vi "SubPanel_PowerConfiguration_Rev11_v2.vi"(8 "error in":errorcluster, 10 "VISAPowerInfoInputArray":T2(array[cluster]), 11 "DCPowerInformationClusterArray_Input":T1(array[cluster])) -> (0 "error out":errorcluster, 2 "VISAPowerInfoOutputArray":T2(array[cluster]), 3 "DCPowerInformationClusterArray_Output":T1(array[cluster]))   [LabVIEW 2019]
panel:
  out "DCPowerInformationClusterArray":T1(array[cluster])
  in  "Update Changes (MUST HAVE ACTIVE CHANNEL SELECTED FOR CHANGES TO BE APPLIED)":bool
  out "VISAPowerInformationClusterArray":T2(array[cluster])
  out "VISAPowerInformationClusterOutput":T3(array[cluster])
  in  "VISAPowerInformationClusterInput":T3(array[cluster])
  in  "Exit SubVI":bool
  in  "Instrument Cards (Must Reconfigure if you add new cards or change the names in NI Max)":T4(tab)=enum."PXIe-4139"
  in  "VISA resource name":refnum<visa-resource-name>
  in  "Apply Power Settings":bool
  out "POWER STATUS":bool
  in  "POWER ON":bool
  in  "Voltage Channel 1":dbl
  in  "Voltage Channel 2":dbl
  in  "Voltage Channel 3":dbl
  in  "Current Limit Channel 1":dbl
  in  "Current Limit Channel 2":dbl
  in  "Current Limit Channel 3":dbl
  out "Parameter Configuration Echo":string[][](array[string])
  out "Configuration Echo":string
  in  "Which Channels to Parallelize":u16(ring) items=["I1+I2", "ALL", "I2+I3"]
  in  "Combination Scheme":u16(ring) items=["OFF", "SERIES", "PARALLEL"]
  in  "voltage level channel 0":dbl format="%.6p"
  in  "voltage level channel 1":dbl format="%.6p"
  in  "voltage level channel 2":dbl format="%.6p"
  in  "voltage level channel 3":dbl format="%.6p"
  in  "voltage level channel 4":dbl format="%.6p"
  in  "voltage level channel 5":dbl format="%.6p"
  in  "voltage level channel 6":dbl format="%.6p"
  in  "voltage level channel 7":dbl format="%.6p"
  in  "voltage level channel 8":dbl format="%.6p"
  in  "voltage level channel 9":dbl format="%.6p"
  in  "voltage level channel 10":dbl format="%.6p"
  in  "voltage level channel 11":dbl format="%.6p"
  in  "voltage level channel 12":dbl format="%.6p"
  in  "voltage level channel 13":dbl format="%.6p"
  in  "voltage level channel 14":dbl format="%.6p"
  in  "voltage level channel 15":dbl format="%.6p"
  in  "voltage level channel 16":dbl format="%.6p"
  in  "voltage level channel 17":dbl format="%.6p"
  in  "voltage level channel 18":dbl format="%.6p"
  in  "voltage level channel 19":dbl format="%.6p"
  in  "voltage level channel 20":dbl format="%.6p"
  in  "voltage level channel 21":dbl format="%.6p"
  in  "voltage level channel 22":dbl format="%.6p"
  in  "voltage level channel 23":dbl format="%.6p"
  in  "Active Channel 0":bool
  in  "Active Channel 1":bool
  in  "Active Channel 2":bool
  in  "Active Channel 3":bool
  in  "Active Channel 4":bool
  in  "Active Channel 5":bool
  in  "Active Channel 6":bool
  in  "Active Channel 7":bool
  in  "Active Channel 8":bool
  in  "Active Channel 9":bool
  in  "Active Channel 10":bool
  in  "Active Channel 11":bool
  in  "Active Channel 12":bool
  in  "Active Channel 13":bool
  in  "Active Channel 14":bool
  in  "Active Channel 15":bool
  in  "Active Channel 16":bool
  in  "Active Channel 17":bool
  in  "Active Channel 18":bool
  in  "Active Channel 19":bool
  in  "Active Channel 20":bool
  in  "Active Channel 21":bool
  in  "Active Channel 22":bool
  in  "Active Channel 23":bool
  in  "Channel Name 0":string="NULL0"
  in  "Channel Name 1":string="1p8V_supply"
  in  "Channel Name 2":string="NULL2"
  in  "Channel Name 3":string="NULL3"
  in  "Channel Name 4":string="NULL4"
  in  "Channel Name 5":string="NULL5"
  in  "Channel Name 6":string="NULL6"
  in  "Channel Name 7":string="NULL7"
  in  "Channel Name 8":string="NULL8"
  in  "Channel Name 9":string="NULL9"
  in  "Channel Name 10":string="NULL10"
  in  "Channel Name 11":string="NULL11"
  in  "Channel Name 12":string="NULL12"
  in  "Channel Name 13":string="NULL13"
  in  "Channel Name 14":string="NULL14"
  in  "Channel Name 15":string="NULL15"
  in  "Channel Name 16":string="NULL16"
  in  "Channel Name 17":string="NULL17"
  in  "Channel Name 18":string="NULL18"
  in  "Channel Name 19":string="NULL19"
  in  "Channel Name 20":string="NULL20"
  in  "Channel Name 21":string="NULL21"
  in  "Channel Name 22":string="NULL22"
  in  "Channel Name 23":string="NULL23"
  in  "Apply Power Settings":bool
  in  "Aperture Time (s)":dbl=0.0001
  in  "Measure Record Length":i32=1000000
  in  "current limit (A)":dbl=0.05
  out "All Channel Numbers Array":string[](array[string])=["0", "1", "2", "3", "4", "5", "6", "7", "8", "9", "10", "11", "12", "13", "14", "15", "16", "17", "18", "19", "20", "21", "22", "23"]
  out "Active Channels Indicator":bool[](array[boolean])
  out "Voltage Array":dbl[](array[numeric])=[1.0, 1.8, 1.2, 1.3, 1.4, 1.5, 1.6, 1.7, 1.8, 1.9, 2.0, 2.1, 2.2, 2.3, 2.4, 2.5, 2.6, 2.7, 2.8, 2.9, 3.0, 3.1, 3.2, 3.3]
  out "Active Channel Numbers Array":string[](array[string])=["1"]
  out "Active Channel Voltage Array":dbl[](array[numeric])=[1.8]
  out "Active Channel Names Array":string[](array[string])=["1p8V_supply"]
  in  "voltage level channel 0":dbl format="%.6p"
  in  "Active Channel 0":bool
  in  "Apply Power Settings":bool
  in  "Channel Name 0":string="1p6_supply"
  out "Active Channel Voltage Array":dbl[](array[numeric])=[1.68]
  out "Active Channels Indicator":bool[](array[boolean])
  out "Voltage Array":dbl[](array[numeric])=[1.68]
  out "Active Channel Names Array":string[](array[string])=["1p6_supply"]
  out "Active Channel Numbers Array":string[](array[string])=["0"]
  out "All Channel Numbers Array":string[](array[string])=["0"]
  in  "current limit (A)":dbl=0.05
  in  "Measure Record Length":i32=1000000
  in  "Aperture Time (s)":dbl=0.001
  out "DCPowerInformationClusterOutput":T5(array[cluster])
  in  "DCPowerInformationClusterInput":T5(array[cluster])
  # "Background Information (Important)\nThis subvi has tabs that allow you to configure different power instruments. There are two options: VISA instruments or DC Power instruments. DC Power instruments are inside of the tester, visa instruments are external. If DCPower instruments are switched out, they will need to be reconfigured within the backend of this code (instructions pending). You are able to identify which channels you want to active, their individual voltage levels and the desired \"name\" of the channel (i.e. if you want channel 0 to be known at the \"ADMV1013_3p3V\" or \"GoodEnough\", you write it here). For the entire instrument, you can determine its capture rate (aperture time) or the current limit. I advise you do NOT alter the \"Measure Record Length\" as this is only if there are issues with the program. Shouldn't ever exceed this value. You apply the settings and they will be echoed back in each tab along with the array above. Multiple instruments can be configured and will show up as separate array elements\n\n\nInstructions (More Important):\n\nSelect instrument of interest (VISA KEITHLEY 2230G-30-6, PXIe-4163, and PXIe-4139 are the ones currently available). \n\n\nFOR DCPOWER INSTRUMENTS (PXI or PXIe)\n\nPress \"Active Channel #\" to select which channels you want to have power applied \n\nType in voltage level in \"Voltage level channel #\"\n\nType in desired channel name in \"Channel Name #\"\n\nType the measurement speed (suggest .0001) in aperture time\n\nType the current limit in \"current limit\"\n\nPress \"Apply Power Settings\" and review the echoed outputs within the tab and in the instrument array above the tabs.\n\nRepeat this process for other instruments\n\n\n\nFOR VISA INSTRUMENTS (NOT PXI or PXIe), note that it is case by case for instruments\n\nSelect resource name (you must know which one it is)\n\nPower on device if using it\n\nApply voltage settings \n\nApply current limits for each channel\n\nSelect which channels you will parallelize if at all\n\nSelect which combination scheme you will apply: OFF (individual channels), SERIES (Channel 1 and 2 in series), PARALLEL (I1 + I2, ALL, I2 + I3)\n\nFOR COMBINATIONS: for a combination scheme you choose, you only apply changes to the first channel of each. example: if you make the system series configuration, you only type you voltage information (i.e. 60V) into channel 1 and the current limit information into channel 1 but channel 3 is still independent of these\n\n\nPress \"Apply Powe Settings\" when complete\n\nReview the echoed values along with the instrument array above"
  # "All Voltage Level Channels are in Volts"
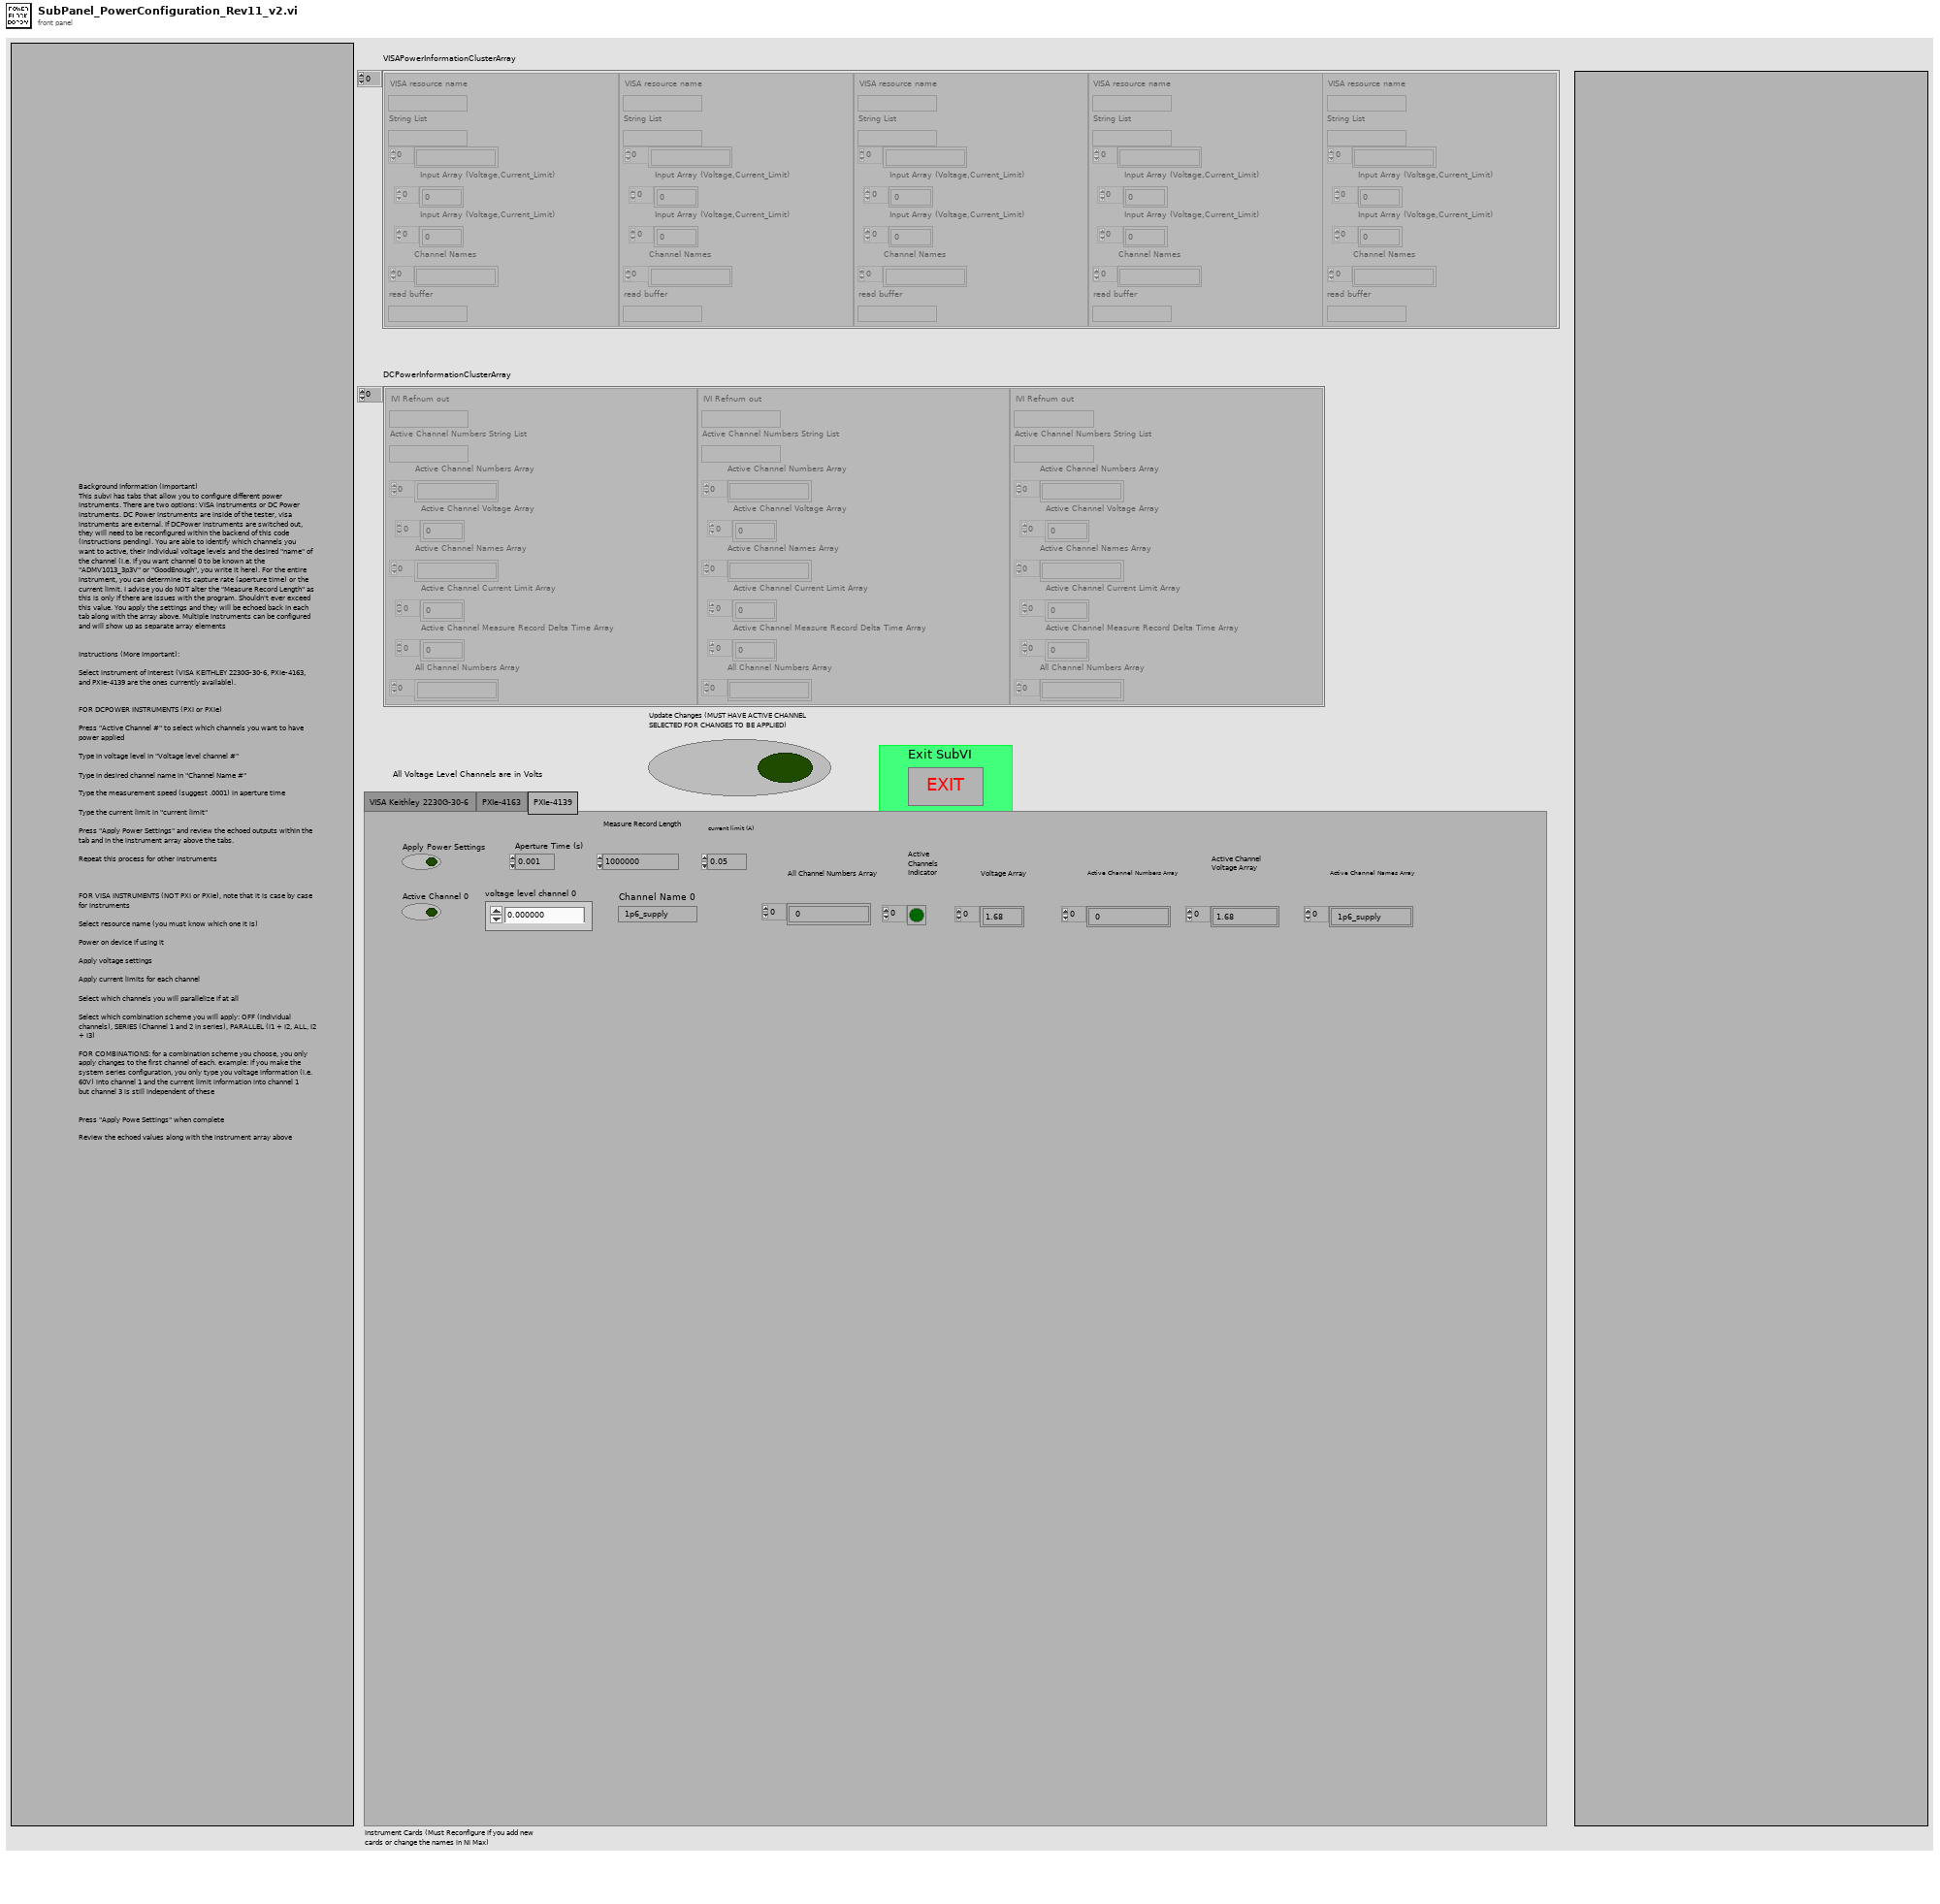
[diagram p1: front panel]
types:
  T1 = cluster{"IVI Refnum out":refnum<k15>, "Active Channel Numbers String List":string, "Active Channel Numbers Array":string[], "Active Channel Voltage Array":dbl[], "Active Channel Names Array":string[], "Active Channel Current Limit Array":dbl[], "Active Channel Measure Record Delta Time Array":dbl[], "All Channel Numbers Array":string[]}[]
  T2 = cluster{"VISA resource name":refnum<visa-resource-name>, "String List":string, string[], "Input Array (Voltage,Current_Limit)":dbl[], "Input Array (Voltage,Current_Limit)":dbl[], "Channel Names":string[], "read buffer":string}[]
  T3 = cluster{"VISA resource name":refnum<visa-resource-name>, "String List":string, string[], "Input Array (Voltage,Current_Limit)":dbl[], "Input Array (Voltage,Current_Limit)":dbl[], "Channel Names":string[]}[]
  T4 = enum32{"VISA Keithley 2230G-30-6", "PXIe-4163", "PXIe-4139"}
  T5 = cluster{"instrument handle out":refnum<k15>, string, string[], dbl[], string[]}[]
  T6 = cluster{"instrument handle out":refnum<k15>, string, string[], dbl[], string[], "Current Limit Output Array":dbl[], dbl[]}[]
  T7 = cluster{"IVI Refnum out":refnum<k15>, "Active Channel Numbers String List":string, "Active Channel Numbers Array":string[], "Active Channel Voltage Array":dbl[], "Active Channel Names Array":string[], "Active Channel Current Limit Array":dbl[], "Active Channel Measure Record Delta Time Array":dbl[], "All Channel Numbers Array":string[]}
  T8 = typedef "VISA_power_Control.ctl" = cluster{"VISA resource name":refnum<visa-resource-name>, "Active Channel List":string, "Active Channel Array":string[], "Input Array (Voltage,Current_Limit)":dbl[], "Input Array (Voltage,Current_Limit)":dbl[], "Channel Names":string[], "read buffer":string, "Channel Names Array":string[]}
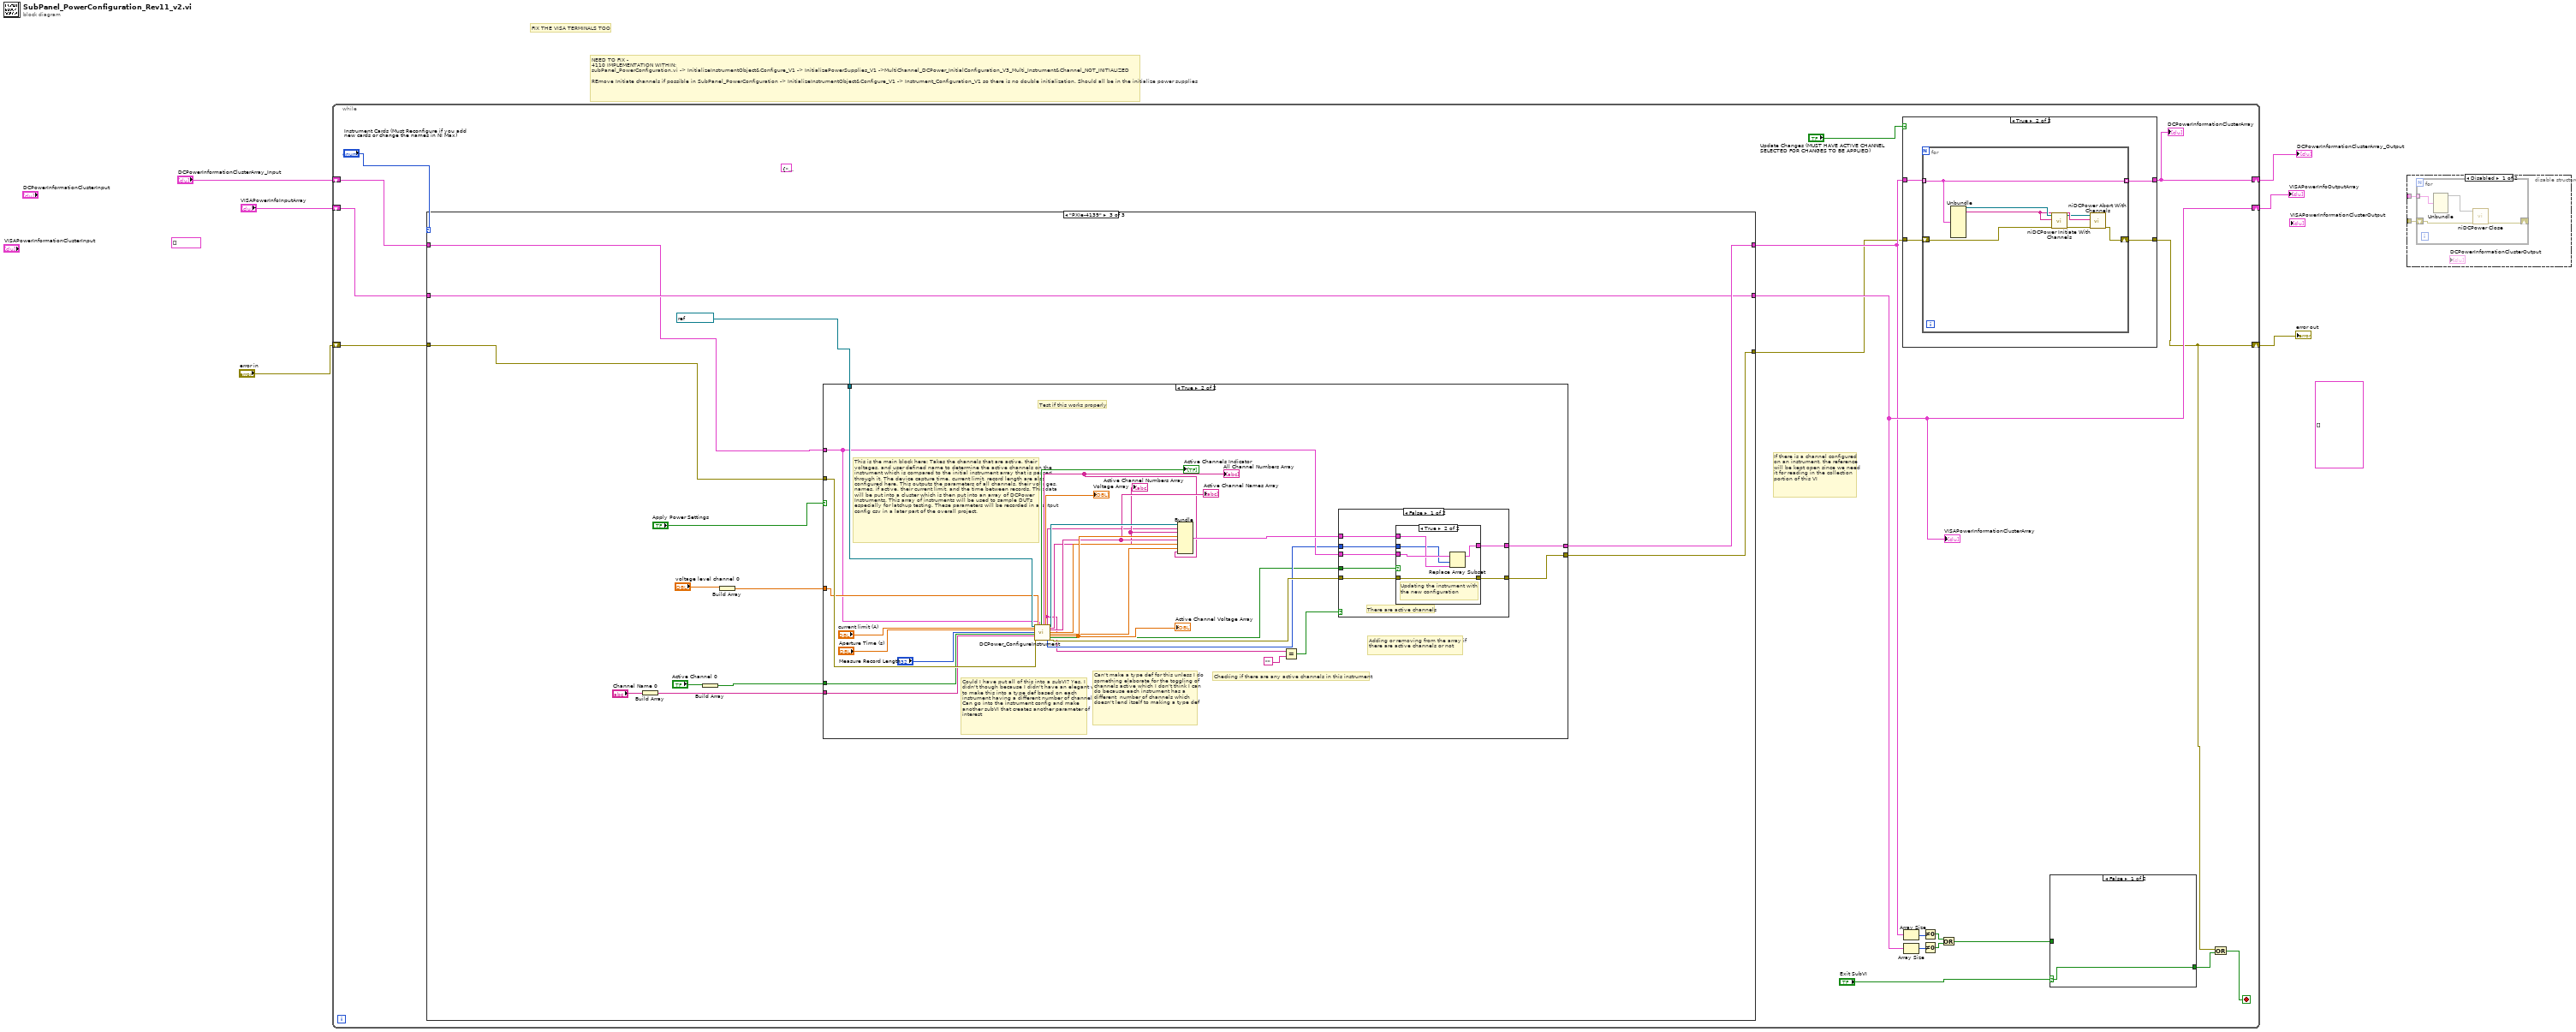
[diagram p0: block diagram]
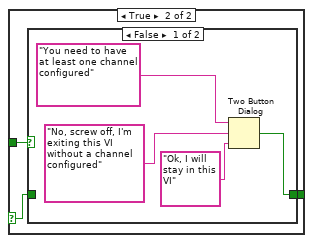
[diagram p4: hidden frame]
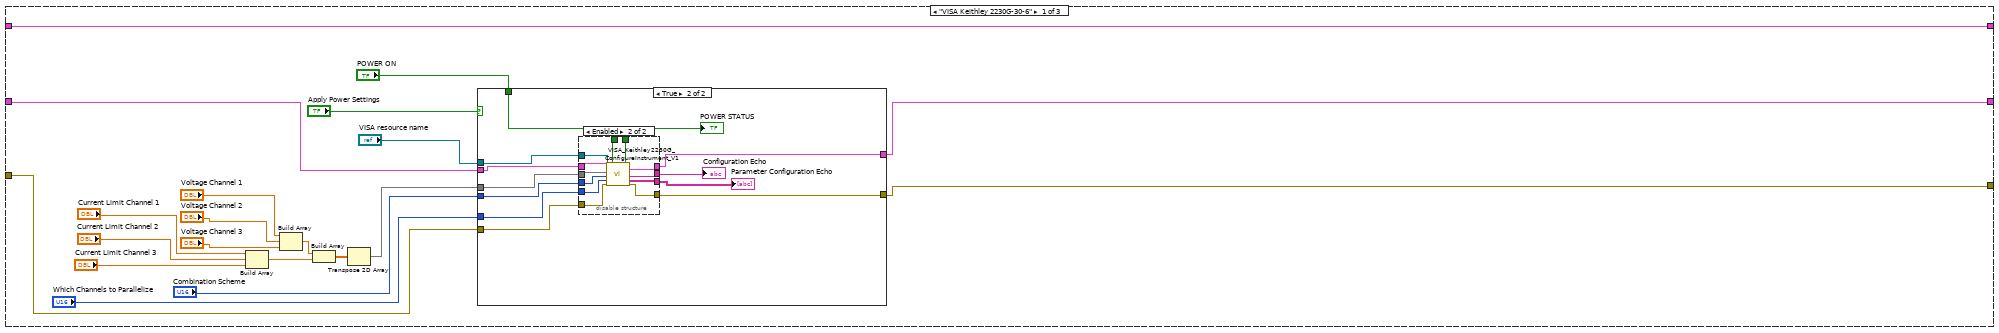
[diagram p6: hidden frame]
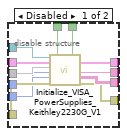
[diagram p8: hidden frame]
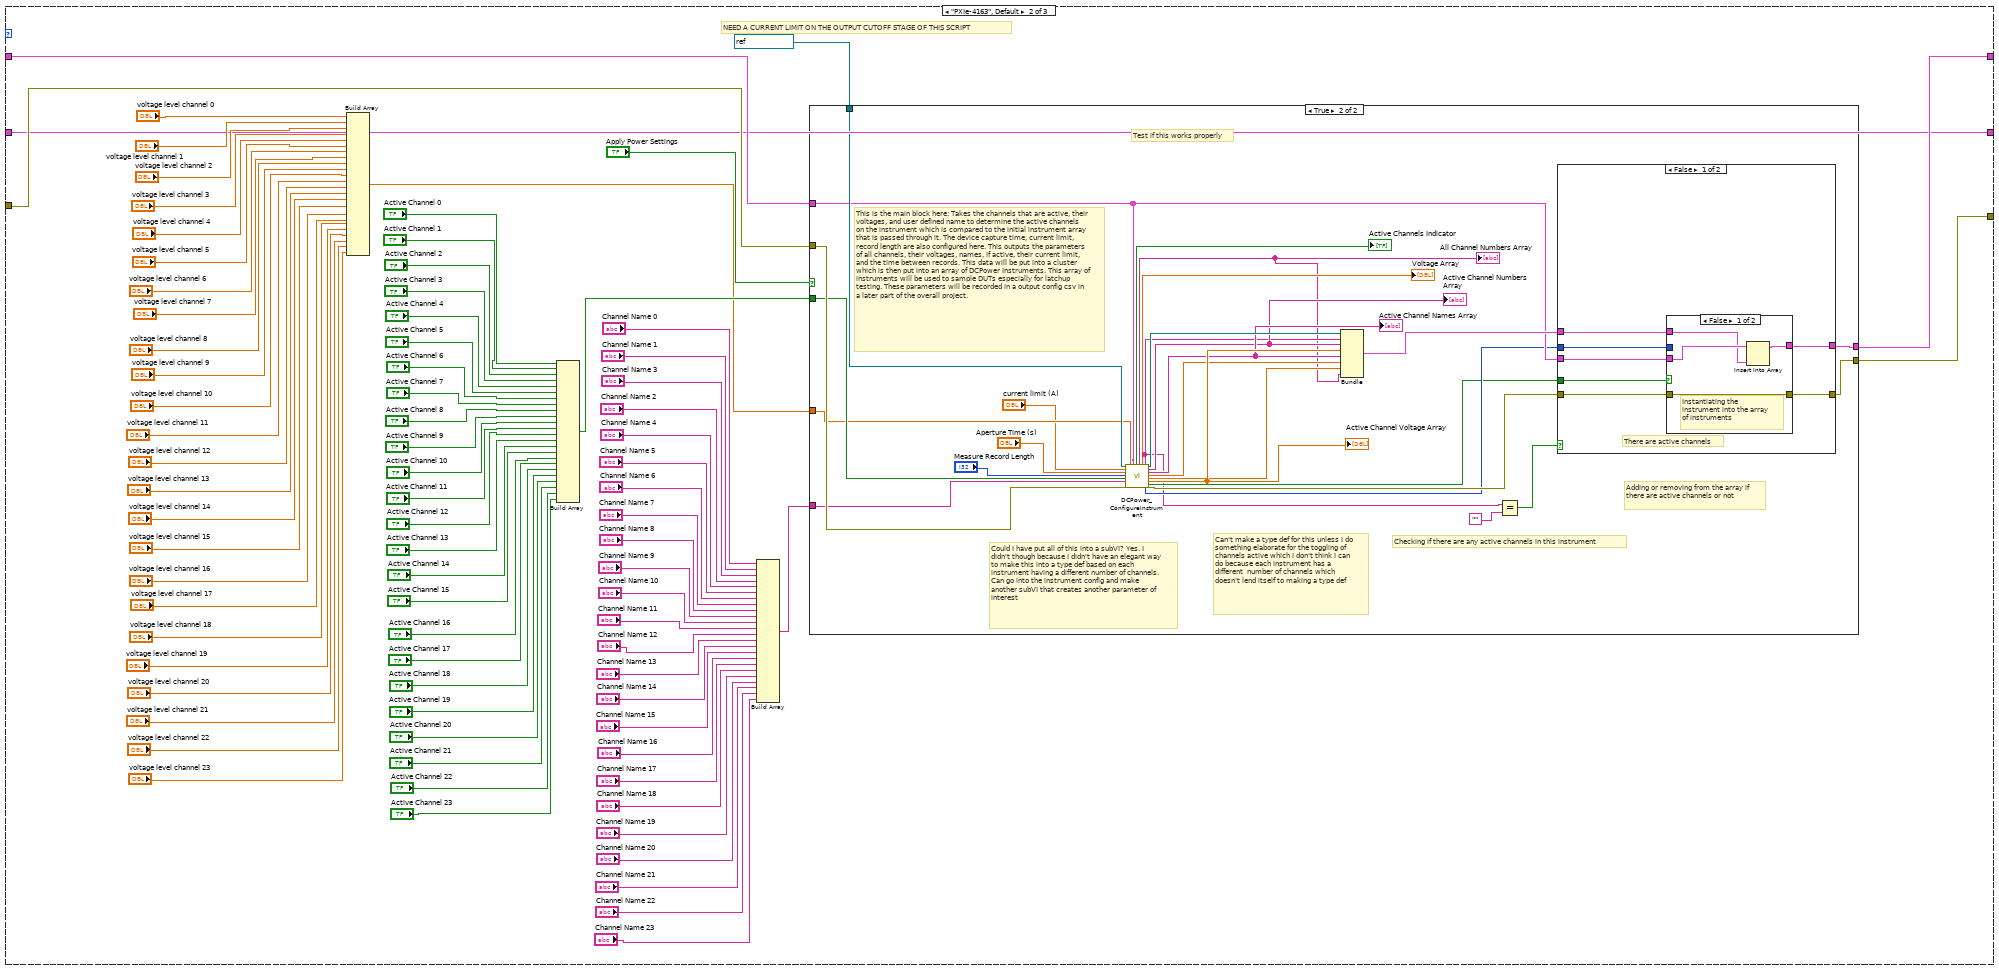
[diagram p9: hidden frame]
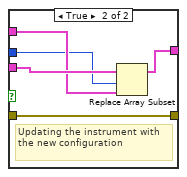
[diagram p11: hidden frame]
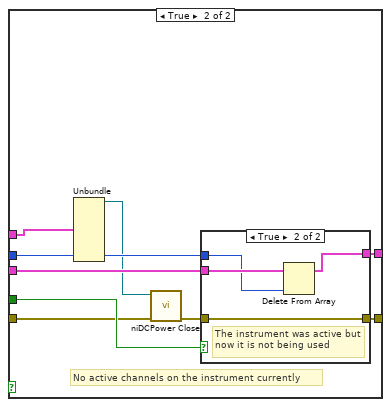
[diagram p12: hidden frame]
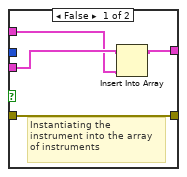
[diagram p15: hidden frame]
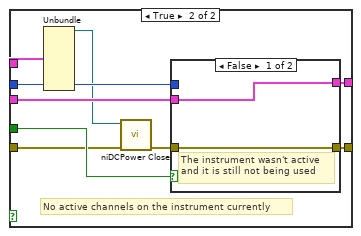
[diagram p16: hidden frame]
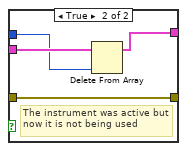
[diagram p17: hidden frame]
diagram:
  (unwired) T1 []
  (unwired) T6 [] ("DCPowerInformationClusterArray_Input")
  # "FIX THE VISA TERMINALS TOO"
  # "NEED TO FIX - \n4110 IMPLEMENTATION WITHIN:\nsubPanel_PowerConfiguration.vi -> InitializeInstrumentObject&Configure_V1 -> InitializePowerSupplies_V1 ->MultiChannel_DCPower_InitialConfiguration_V3_Multi_Instrument&Channel_NOT_INITIALIZED\n\nREmove Initiate channels if possible in SubPanel_PowerConfiguration -> InitializeInstrumentObject&Configure_V1 -> Instrument_Configuration_V1 so there is no double initialization. Should all be in the initialize power supplies"
  n1 = while {
    shift-right: [w11] -> w2
    shift-left: "DCPowerInformationClusterArray_Input" -> [w24]
    shift-right: [w7] -> w5
    shift-left: "error in" -> [w23]
    shift-right: [w20] -> w3
    shift-left: "VISAPowerInfoInputArray" -> [w21]
    stop <- w12 stop-if-true
    (unwired) T7 {"IVI Refnum out"="", "Active Channel Numbers String List"="", "Active Channel Numbers Array"=[], "Active Channel Voltage Array"=[], "Active Channel Names Array"=[], "Active Channel Current Limit Array"=[], "Active Channel Measure Record Delta Time Array"=[], "All Channel Numbers Array"=[]} ("output cluster")
    # "If there is a channel configured on an instrument, the reference will be kept open since we need it for reading in the collection portion of this VI"
    n2 = case shown="\"PXIe-4139\"" "Instrument Cards (Must Reconfigure if you add new cards or change the names in NI Max)" {
      tunnel: w24 -> [w63 w113 w247]
      tunnel: w23 -> [w51 w109 w255]
      tunnel: [w48 w108 w249] -> w8
      tunnel: [w63 w107 w250] -> w10
      tunnel: w21 -> [w64 w106 w248]
      tunnel: [w47 w106 w248] -> w20
      frame "VISA Keithley 2230G-30-6" {
        n3 = Build Array("Current Limit Channel 1", "Current Limit Channel 2", "Current Limit Channel 3") -> (w61:dbl[])
        n4 = Build Array("Voltage Channel 1", "Voltage Channel 2", "Voltage Channel 3") -> (w60:dbl[])
        n5 = Build Array(w60, w61) -> (w62:dbl[][])
        n6 = Transpose 2D Array(2D array=w62) -> (transposed array=w52:dbl[][])
        n7 = case shown="True" "Apply Power Settings" {
          tunnel: "VISA resource name" -> [_ w80]
          tunnel: w64 -> [w67 w79]
          tunnel: "POWER ON" -> [_ w78]
          tunnel: w52 -> [_ w77]
          tunnel: w51 -> [w68 w76]
          tunnel: "Which Channels to Parallelize" -> [_ w75]
          tunnel: "Combination Scheme" -> [_ w74]
          tunnel: [w67 w70] -> w47
          tunnel: [w68 w69] -> w48
          frame False {
          }
          frame True {
            n8 = disable-structure shown="Enabled" {
              disable-tunnel: w80 -> [w92 w102]
              disable-tunnel: w79 -> [w91 w101]
              disable-tunnel: w78 -> [w90 w103]
              disable-tunnel: w77 -> [w89 w100]
              disable-tunnel: w76 -> [w88 w97]
              disable-tunnel: w75 -> [w87 w98]
              disable-tunnel: w74 -> [w86 w99]
              disable-tunnel: [w85 w104] -> w73
              disable-tunnel: [w84 w95] -> w72
              disable-tunnel: [w83 w94] -> w71
              disable-tunnel: [w82 w96] -> w70
              disable-tunnel: [w81 w93] -> w69
              frame Disabled {
                n9 = call "Initialize_VISA_PowerSupplies_Keithley2230G_V1.vi"("VISA resource name"=w92, "VISAPowerInfoInputArray"=w91, "Input Array (Voltage,Current_Limit)"=w89, "Combination Scheme"=w86, "Which Channels to Parallelize"=w87, "error in"=w88, "POWER STATUS IN"=w90) -> ("POWER STATUS OUT"=w85:bool, "VISAPowerInfoOutputArray"=w82:T2, "Configuration Echo"=w84:string, "Parameter Configuration Echo"=w83:string[][], "error out"=w81:errorcluster)  [unwired: 8 in]
              }
              frame Enabled {
                n10 = call "VISA_Keithley2230G_ConfigureInstrument_V1.vi"("VISA resource name"=w102, "VISAPowerInfoInputArray"=w101, "Input Array (Voltage,Current_Limit)"=w100, "Combination Scheme"=w99, "Which Channels to Parallelize"=w98, "error in"=w97, "POWER STATUS IN"=w103) -> ("POWER STATUS OUT"=w104:bool, "VISAPowerInfoOutputArray"=w96:T8[], "Configuration Echo"=w95:string, "Parameter Configuration Echo"=w94:string[][], "error out"=w93:errorcluster)  [unwired: 8 in]
              }
            }
            "POWER STATUS" <- w73
            "Configuration Echo" <- w72
            "Parameter Configuration Echo" <- w71
          }
        }
      }
      frame "PXIe-4163", Default {
        # "NEED A CURRENT LIMIT ON THE OUTPUT CUTOFF STAGE OF THIS SCRIPT"
        n11 = Build Array("voltage level channel 0", "voltage level channel 1", "voltage level channel 2", "voltage level channel 3", "voltage level channel 4", "voltage level channel 5", "voltage level channel 6", "voltage level channel 7", "voltage level channel 8", "voltage level channel 9", "voltage level channel 10", "voltage level channel 11", "voltage level channel 12", "voltage level channel 13", "voltage level channel 14", "voltage level channel 15", "voltage level channel 16", "voltage level channel 17", "voltage level channel 18", "voltage level channel 19", "voltage level channel 20", "voltage level channel 21", "voltage level channel 22", "voltage level channel 23") -> (w105:dbl[])
        n12 = Build Array("Active Channel 0", "Active Channel 1", "Active Channel 2", "Active Channel 3", "Active Channel 4", "Active Channel 5", "Active Channel 6", "Active Channel 7", "Active Channel 8", "Active Channel 9", "Active Channel 10", "Active Channel 11", "Active Channel 12", "Active Channel 13", "Active Channel 14", "Active Channel 15", "Active Channel 16", "Active Channel 17", "Active Channel 18", "Active Channel 19", "Active Channel 20", "Active Channel 21", "Active Channel 22", "Active Channel 23") -> (w111:bool[])
        n13 = Build Array("Channel Name 0", "Channel Name 1", "Channel Name 3", "Channel Name 2", "Channel Name 4", "Channel Name 5", "Channel Name 6", "Channel Name 7", "Channel Name 8", "Channel Name 9", "Channel Name 10", "Channel Name 11", "Channel Name 12", "Channel Name 13", "Channel Name 14", "Channel Name 15", "Channel Name 16", "Channel Name 17", "Channel Name 18", "Channel Name 19", "Channel Name 20", "Channel Name 21", "Channel Name 22", "Channel Name 23") -> (w110:string[])
        n14 = case shown="True" "Apply Power Settings" {
          tunnel: w113 -> [w188 w198]
          tunnel: refnum<k15> "PXIe-4163" ("resource name") -> [_ w215]
          tunnel: w111 -> [_ w213]
          tunnel: w110 -> [_ w211]
          tunnel: w109 -> [w187 w214]
          tunnel: [w187 w196] -> w108
          tunnel: [w188 w195] -> w107
          tunnel: w105 -> [_ w212]
          frame False {
          }
          frame True {
            # "This is the main block here: Takes the channels that are active, their voltages, and user defined name to determine the active channels on the instrument which is compared to the initial instrument array that is passed through it. The device capture time, current limit, record length are also configured here. This outputs the parameters of all channels, their voltages, names, if active, their current limit, and the time between records. This data will be put into a cluster which is then put into an array of DCPower Instruments. This array of instruments will be used to sample DUTs especially for latchup testing. These parameters will be recorded in a output config csv in a later part of the overall project."
            # "Checking if there are any active channels in this instrument"
            # "Adding or removing from the array if there are active channels or not"
            # "Could I have put all of this into a subVI? Yes. I didn't though because I didn't have an elegant way to make this into a type def based on each instrument having a different number of channels. Can go into the instrument config and make another subVI that creates another parameter of interest"
            # "Can't make a type def for this unless I do something elaborate for the toggling of channels active which I don't think I can do because each instrument has a different  number of channels which doesn't lend itself to making a type def"
            # "Test if this works properly"
            n15 = call "DCPower_ConfigureInstrument.vi"("IVI Refnum in"=w215, "current limit"="current limit (A)", "Aperture Time"="Aperture Time (s)", "Measure Record Length"="Measure Record Length", "Active Channels Input"=w213, "Channel Name Array"=w211, "error in (no error)"=w214, "Voltage Array Input"=w212, "DCPowerInformationClusterArray_Input"=w198) -> ("Active Channels Indicator"=→"Active Channels Indicator":bool[], "All Channel Numbers Array"=w189:string[], "Total Voltage Indicator Array"=→"Voltage Array":dbl[], "Active Channel Numbers String List"=w190:string, "IVI Ref index"=w194:i32, "IVI Refnum out"=w206:refnum<k15>, "Active Channel Numbers Array"=w192:string[], "Active Channel Names Array"=w204:string[], "Active Channel Current Limit Array"=w203:dbl[], "Active Channel Measure Record Delta Time Array"=w202:dbl[], "Active Channel Voltage Array"=w205:dbl[], "IVI Ref Present?"=w193:bool, "error out"=w197:errorcluster)  [unwired: 3 in, 3 out]
            "All Channel Numbers Array" <- w189
            "Active Channel Numbers Array" <- w192
            "Active Channel Names Array" <- w204
            "Active Channel Voltage Array" <- w205
            n16 = Bundle("IVI Refnum out"=w206, "Active Channel Numbers String List"=w190, "Active Channel Numbers Array"=w192, "Active Channel Voltage Array"=w205, "Active Channel Names Array"=w204, "Active Channel Current Limit Array"=w203, "Active Channel Measure Record Delta Time Array"=w202, "All Channel Numbers Array"=w189) -> (w199:T7)  [unwired: 1 in]
            n17 = Equal?(x=w190, y="") -> (x = y?=w200:bool)
            n18 = case shown="False" w200 {
              tunnel: w193 -> [w222 w239]
              tunnel: [w221 w236] -> w195
              tunnel: [w220 w237] -> w196
              tunnel: w197 -> [w219 w234]
              tunnel: w194 -> [w218 w238]
              tunnel: w199 -> [w217 w232]
              tunnel: w198 -> [w216 w240]
              frame False {
                # "There are active channels"
                n19 = case shown="False" w222 {
                  tunnel: w216 -> [w225 w231]
                  tunnel: w217 -> [w224 w230]
                  tunnel: w218 -> [_ w229]
                  tunnel: w219 -> [w226 w228]
                  tunnel: [w226 w228] -> w220
                  tunnel: [w223 w227] -> w221
                  frame False {
                    # "Instantiating the instrument into the array of instruments"
                    n20 = Insert Into Array(array=w225, new element=w224) -> (w223:T1)  [unwired: 1 in]
                  }
                  frame True {
                    # "Updating the instrument with the new configuration"
                    n21 = Replace Array Subset(array=w231, new element=w230, index=w229) -> (w227:T1)
                  }
                }
              }
              frame True {
                # "No active channels on the instrument currently"
                n22 = Unbundle(w232) -> ("IVI Refnum out"=w235:refnum<k15>)  [unwired: 7 out]
                n23 = call <instrlib>:"niDCPower Close.vi"("error in (no error)"=w234, "instrument handle"=w235) -> ("error out"=w233:errorcluster)  [unwired: 9 in]
                n24 = case shown="True" w239 {
                  tunnel: w240 -> [w242 w246]
                  tunnel: w238 -> [_ w245]
                  tunnel: [w241 w244] -> w237
                  tunnel: w233 -> [w241 w244]
                  tunnel: [w242 w243] -> w236
                  frame False {
                    # "The instrument wasn't active and it is still not being used"
                  }
                  frame True {
                    # "The instrument was active but now it is not being used"
                    n25 = Delete From Array(array=w246, index=w245) -> (array with subset deleted=w243:T1)  [unwired: 1 in, 1 out]
                  }
                }
              }
            }
          }
        }
      }
      frame "PXIe-4139" {
        n26 = Build Array("Channel Name 0") -> (w252:string[])
        n27 = Build Array("Active Channel 0") -> (w253:bool[])
        n28 = Build Array("voltage level channel 0") -> (w254:dbl[])
        n29 = case shown="True" "Apply Power Settings" {
          tunnel: w247 -> [w261 w271]
          tunnel: refnum<k15> "PXI-4139" ("resource name") -> [_ w288]
          tunnel: w253 -> [_ w286]
          tunnel: w252 -> [_ w284]
          tunnel: w255 -> [w260 w287]
          tunnel: [w260 w269] -> w249
          tunnel: [w261 w268] -> w250
          tunnel: w254 -> [_ w285]
          frame False {
          }
          frame True {
            # "This is the main block here: Takes the channels that are active, their voltages, and user defined name to determine the active channels on the instrument which is compared to the initial instrument array that is passed through it. The device capture time, current limit, record length are also configured here. This outputs the parameters of all channels, their voltages, names, if active, their current limit, and the time between records. This data will be put into a cluster which is then put into an array of DCPower Instruments. This array of instruments will be used to sample DUTs especially for latchup testing. These parameters will be recorded in a output config csv in a later part of the overall project."
            # "Checking if there are any active channels in this instrument"
            # "Adding or removing from the array if there are active channels or not"
            # "Could I have put all of this into a subVI? Yes. I didn't though because I didn't have an elegant way to make this into a type def based on each instrument having a different number of channels. Can go into the instrument config and make another subVI that creates another parameter of interest"
            # "Can't make a type def for this unless I do something elaborate for the toggling of channels active which I don't think I can do because each instrument has a different  number of channels which doesn't lend itself to making a type def"
            # "Test if this works properly"
            n30 = call "DCPower_ConfigureInstrument.vi"("IVI Refnum in"=w288, "current limit"="current limit (A)", "Aperture Time"="Aperture Time (s)", "Measure Record Length"="Measure Record Length", "Active Channels Input"=w286, "Channel Name Array"=w284, "error in (no error)"=w287, "Voltage Array Input"=w285, "DCPowerInformationClusterArray_Input"=w271) -> ("Active Channels Indicator"=→"Active Channels Indicator":bool[], "All Channel Numbers Array"=w262:string[], "Total Voltage Indicator Array"=→"Voltage Array":dbl[], "Active Channel Numbers String List"=w263:string, "IVI Ref index"=w267:i32, "IVI Refnum out"=w279:refnum<k15>, "Active Channel Numbers Array"=w265:string[], "Active Channel Names Array"=w277:string[], "Active Channel Current Limit Array"=w276:dbl[], "Active Channel Measure Record Delta Time Array"=w275:dbl[], "Active Channel Voltage Array"=w278:dbl[], "IVI Ref Present?"=w266:bool, "error out"=w270:errorcluster)  [unwired: 3 in, 3 out]
            "All Channel Numbers Array" <- w262
            "Active Channel Numbers Array" <- w265
            "Active Channel Names Array" <- w277
            "Active Channel Voltage Array" <- w278
            n31 = Bundle("IVI Refnum out"=w279, "Active Channel Numbers String List"=w263, "Active Channel Numbers Array"=w265, "Active Channel Voltage Array"=w278, "Active Channel Names Array"=w277, "Active Channel Current Limit Array"=w276, "Active Channel Measure Record Delta Time Array"=w275, "All Channel Numbers Array"=w262) -> (w272:T7)  [unwired: 1 in]
            n32 = Equal?(x=w263, y="") -> (x = y?=w273:bool)
            n33 = case shown="False" w273 {
              tunnel: w266 -> [w295 w312]
              tunnel: [w294 w309] -> w268
              tunnel: [w293 w310] -> w269
              tunnel: w270 -> [w292 w307]
              tunnel: w267 -> [w291 w311]
              tunnel: w272 -> [w290 w305]
              tunnel: w271 -> [w289 w313]
              frame False {
                # "There are active channels"
                n34 = case shown="True" w295 {
                  tunnel: w289 -> [w298 w304]
                  tunnel: w290 -> [w297 w303]
                  tunnel: w291 -> [_ w302]
                  tunnel: w292 -> [w299 w301]
                  tunnel: [w299 w301] -> w293
                  tunnel: [w296 w300] -> w294
                  frame False {
                    # "Instantiating the instrument into the array of instruments"
                    n35 = Insert Into Array(array=w298, new element=w297) -> (w296:T1)  [unwired: 1 in]
                  }
                  frame True {
                    # "Updating the instrument with the new configuration"
                    n36 = Replace Array Subset(array=w304, new element=w303, index=w302) -> (w300:T1)
                  }
                }
              }
              frame True {
                # "No active channels on the instrument currently"
                n37 = Unbundle(w305) -> ("IVI Refnum out"=w308:refnum<k15>)  [unwired: 7 out]
                n38 = call <instrlib>:"niDCPower Close.vi"("error in (no error)"=w307, "instrument handle"=w308) -> ("error out"=w306:errorcluster)  [unwired: 9 in]
                n39 = case shown="False" w312 {
                  tunnel: w313 -> [w315 w319]
                  tunnel: w311 -> [_ w318]
                  tunnel: [w314 w317] -> w310
                  tunnel: w306 -> [w314 w317]
                  tunnel: [w315 w316] -> w309
                  frame False {
                    # "The instrument wasn't active and it is still not being used"
                  }
                  frame True {
                    # "The instrument was active but now it is not being used"
                    n40 = Delete From Array(array=w319, index=w318) -> (array with subset deleted=w316:T1)  [unwired: 1 in, 1 out]
                  }
                }
              }
            }
          }
        }
      }
    }
    "VISAPowerInformationClusterArray" <- w20
    n41 = case shown="True" "Update Changes (MUST HAVE ACTIVE CHANNEL SELECTED FOR CHANGES TO BE APPLIED)" {
      tunnel: [w25 w29] -> w11
      tunnel: w10 -> [w25 w30]
      tunnel: w8 -> [w26 w28]
      tunnel: [w26 w27] -> w7
      frame False {
      }
      frame True {
        n42 = for {
          tunnel: [w37] -> w29 mode=indexing
          tunnel: w30 -> [w37] mode=indexing
          shift-right: [w33] -> w27
          shift-left: w28 -> [w35]
          n43 = Unbundle(w37) -> ("IVI Refnum out"=w36:refnum<k15>, "Active Channel Numbers String List"=w32:string)  [unwired: 6 out]
          n44 = call <instrlib>:"niDCPower Initiate With Channels.vi"("error in (no error)"=w35, "channel name"=w32, "instrument handle"=w36) -> ("error out"=w34:errorcluster, "instrument handle out"=w31:refnum<k15>)  [unwired: 7 in]
          n45 = call <instrlib>:"niDCPower Abort With Channels.vi"("error in (no error)"=w34, "channel name"=w32, "instrument handle"=w31) -> ("error out"=w33:errorcluster)  [unwired: 7 in, 1 out]
        }
      }
    }
    "DCPowerInformationClusterArray" <- w11
    n46 = Array Size(array=w10) -> (size(s)=w19:i32)
    n47 = Array Size(array=w20) -> (size(s)=w18:i32)
    n48 = Not Equal To 0?(x=w19) -> (x != 0?=w16:bool)
    n49 = Not Equal To 0?(x=w18) -> (x != 0?=w17:bool)
    n50 = Or(x=w16, y=w17) -> (x .or. y?=w14:bool)
    n51 = case shown="False" "Exit SubVI" {
      selector: "Exit SubVI" -> [w38 w39]
      tunnel: w14 -> [_ w41]
      tunnel: [w38 w40] -> w13
      frame False {
      }
      frame True {
        n52 = case shown="False" w41 {
          tunnel: [w43 w46] -> w40
          tunnel: w39 -> [_ w46]
          frame False {
            n53 = Two Button Dialog(message="You need to have at least one channel configured", 1:"Ok, I will stay in this VI" ("F button name (\"Cancel\")"), 2:"No, screw off, I'm exiting this VI without a channel configured" ("T button name (\"OK\")")) -> (T button?=w43:bool)
          }
          frame True {
          }
        }
      }
    }
    n54 = Or(x=w7, y=w13) -> (x .or. y?=w12:bool)
  }
  "error out" <- w5
  "VISAPowerInfoOutputArray" <- w3
  "DCPowerInformationClusterArray_Output" <- w2
  n55 = disable-structure shown="Disabled" {
    disable-tunnel: _ -> [w321 _]
    disable-tunnel: _ -> [w320 _]
    frame Disabled {
      n56 = for {
        shift-right: [w322] -> _
        shift-left: w321 -> [w325]
        tunnel: w320 -> [w324] mode=indexing
        n57 = Unbundle(w324) -> ("instrument handle out"=w323)  [unwired: 4 out]
        n58 = call <instrlib>:"niDCPower Close.vi"("error in (no error)"=w325, "instrument handle"=w323) -> ("error out"=w322:errorcluster)  [unwired: 9 in]
      }
    }
    frame Enabled {
    }
  }
